vi "CIC length.vi"(11 "CIC total length":u16) -> (2 "Length extend":u8, 3 "CIC length":u16)   [LabVIEW 2020]
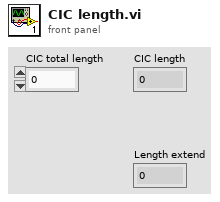
[diagram p1: front panel]
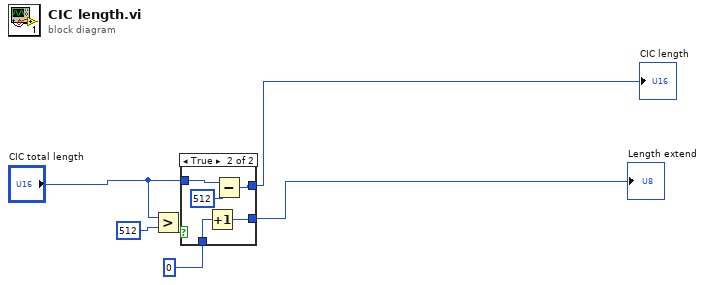
[diagram p0: block diagram]
diagram:
  n1 = Greater?(x="CIC total length", y=u16 512) -> (0:w1:bool)
  n2 = case shown="True" w1 {
    tunnel: "CIC total length" -> [w8 w13]
    tunnel: u8 0 -> [w7 w12]
    tunnel: [w8 w11] -> w5
    tunnel: [w7 w10] -> w6
    frame False {
    }
    frame True {
      n3 = Increment(x=w12) -> (x+1=w10:u8)
      n4 = Subtract(x=w13, y=u16 512) -> (x-y=w11:u16)
    }
  }
  "Length extend" <- w6
  "CIC length" <- w5
